vi "zad3.vi"() -> ()   [LabVIEW 2025]
panel:
  out "Output Pages":i32[](array[numeric])
  in  "Input Pages":string
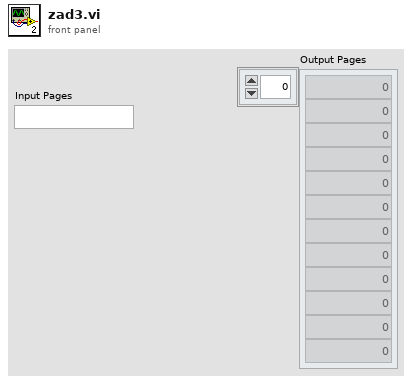
[diagram p1: front panel]
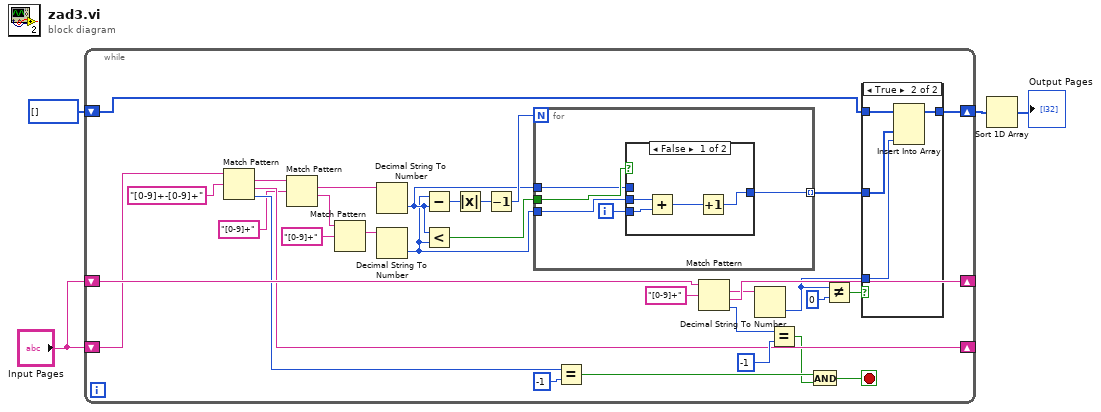
[diagram p0: block diagram]
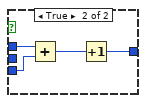
[diagram p3: hidden frame]
diagram:
  n1 = while {
    shift-right: [w31] -> _
    shift-left: "Input Pages" -> [w32]
    shift-right: [w29] -> _
    shift-left: "Input Pages" -> [w30]
    shift-right: [w9] -> w2
    shift-left: i32[] [] -> [w10]
    stop <- w24 stop-if-true
    n2 = Match Pattern(string=w30, regular expression="[0-9]+-[0-9]+") -> (match substring=w23:string, after substring=w29:string, offset past match=w27:i32)  [unwired: 1 in, 1 out]
    n3 = Match Pattern(string=w23, regular expression="[0-9]+") -> (match substring=w15:string, after substring=w20:string)  [unwired: 1 in, 2 out]
    n4 = Match Pattern(string=w20, regular expression="[0-9]+") -> (match substring=w12:string)  [unwired: 1 in, 3 out]
    n5 = Decimal String To Number(string=w15) -> (number=w14:i32)  [unwired: 2 in, 1 out]
    n6 = Decimal String To Number(string=w12) -> (number=w13:i32)  [unwired: 2 in, 1 out]
    n7 = Subtract(x=w13, y=w14) -> (x-y=w19:i32)
    n8 = Less?(x=w14, y=w13) -> (x < y?=w18:bool)
    n9 = Absolute Value(x=w19) -> (abs(x)=w17:i32)
    n10 = Decrement(x=w17) -> (x-1=w16:i32)
    n11 = for {
      N: w16 -> [_]
      tunnel: w18 -> [w46]
      tunnel: w14 -> [w45]
      tunnel: w13 -> [w43]
      tunnel: [w42] -> w5 mode=indexing
      i -> [w44]
      n12 = case shown="False" w46 {
        tunnel: w45 -> [_ w54]
        tunnel: w44 -> [w48 w53]
        tunnel: [w47 w51] -> w42
        tunnel: w43 -> [w49 _]
        frame False {
          n13 = Add(x=w49, y=w48) -> (x+y=w50:i32)
          n14 = Increment(x=w50) -> (x+1=w47:i32)
        }
        frame True {
          n15 = Add(x=w54, y=w53) -> (x+y=w52:i32)
          n16 = Increment(x=w52) -> (x+1=w51:i32)
        }
      }
    }
    n17 = Equal?(x=w27, y=-1) -> (x = y?=w26:bool)
    n18 = Match Pattern(string=w32, regular expression="[0-9]+") -> (match substring=w11:string, after substring=w31:string, offset past match=w34:i32)  [unwired: 1 in, 1 out]
    n19 = Decimal String To Number(string=w11) -> (number=w8:i32)  [unwired: 2 in, 1 out]
    n20 = Equal?(x=w34, y=-1) -> (x = y?=w25:bool)
    n21 = And(x=w26, y=w25) -> (x .and. y?=w24:bool)
    n22 = Not Equal?(x=w8, y=0) -> (x != y?=w6:bool)
    n23 = case shown="True" w6 {
      tunnel: w10 -> [w37 w39]
      tunnel: w5 -> [_ w38]
      tunnel: w8 -> [_ w41]
      tunnel: [w37 w40] -> w9
      frame False {
      }
      frame True {
        n24 = Insert Into Array(array=w39, new element #1=w38, new element #2=w41) -> (w40:i32[])  [unwired: 1 in]
      }
    }
  }
  n25 = Sort 1D Array(array=w2) -> (sorted array=→"Output Pages":i32[])
